vi "GV-ZoomWindowDrag.vi"(6 "Y":dbl, 7 "Gviewer in":refnum<class "Gviewer.lvclass">, 8 "error in (no error)":errorcluster, 10 "Coords":T1, 11 "pict in":picture) -> (0 "error out":errorcluster, 3 "pict out":picture)   [LabVIEW 2020, in "Sgraph_lib_V1.lvlib" / "Gviewer.lvclass"]
doc: "Andre Koelewijn, 1 May 2021\n\nDraw the zoom window"
uses:
  Gviewer.lvclass
  <vilib>/Utility/miscctls.llb/LVPoint32TypeDef.ctl
  Gviewer.lvclass/Gviewer.ctl
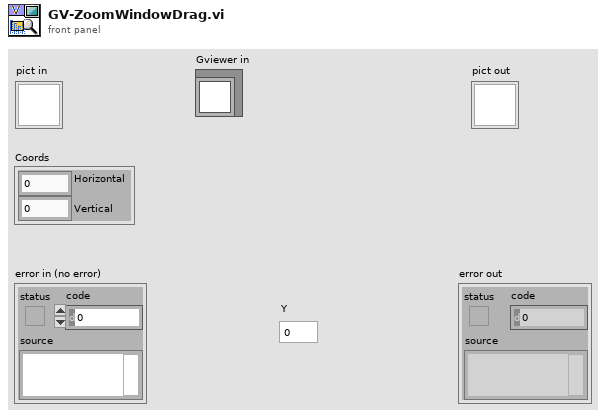
[diagram p1: front panel]
types:
  T1 = typedef "LVPoint32TypeDef.ctl" = cluster{"Horizontal":i32, "Vertical":i32}
  T2 = cluster{"Width":i16, "Style":enum32{"Solid", "Dash", "Dot", "DashDot", "DashDotDot"}}
  T3 = cluster{"left":i16, "top":i16, "right":i16, "bottom":i16}
  T4 = cluster{"horizontal":enum16{"left", "center", "right"}, "vertical":enum16{"top", "center", "bottom"}}
  T5 = typedef "Sgraph_lib_V1.lvlib/Gviewer.lvclass/Typedef_SelProperties.ctl" = cluster{"Color":u32, "LineType":T6, "max":dbl, "min":dbl}
  T6 = typedef "Sgraph_lib_V1.lvlib/Gviewer.lvclass/Typedef_LineType.ctl" = enum16{"num_bare", "num_MinMax_Area", "num_MinMax_Lines", "num_MinMax_Forfor", "num_Max_Area", "num_Max_Line", "num_Max_Forfor", "num_Min_Area", "num_Min_Line", "num_Min_Fosfor", "Boolean_Line_01", "Boolean_Area_01", "Boolean_Fosfor_01", "Boolean_Line_TF", "Boolean_Area_TF", "Boolean_Fosfor_TF", "Boolean_OnOff_Line", "Boolean_OnOff_Area", "Boolean_OnOff_Fosfor", "Boolean_spare", "StringEvent_Line", "StringEvent_TimeLine"}
  T7 = typedef "LVRectTypeDef.ctl" = cluster{"Left":i16, "Top":i16, "Right":i16, "Bottom":i16}
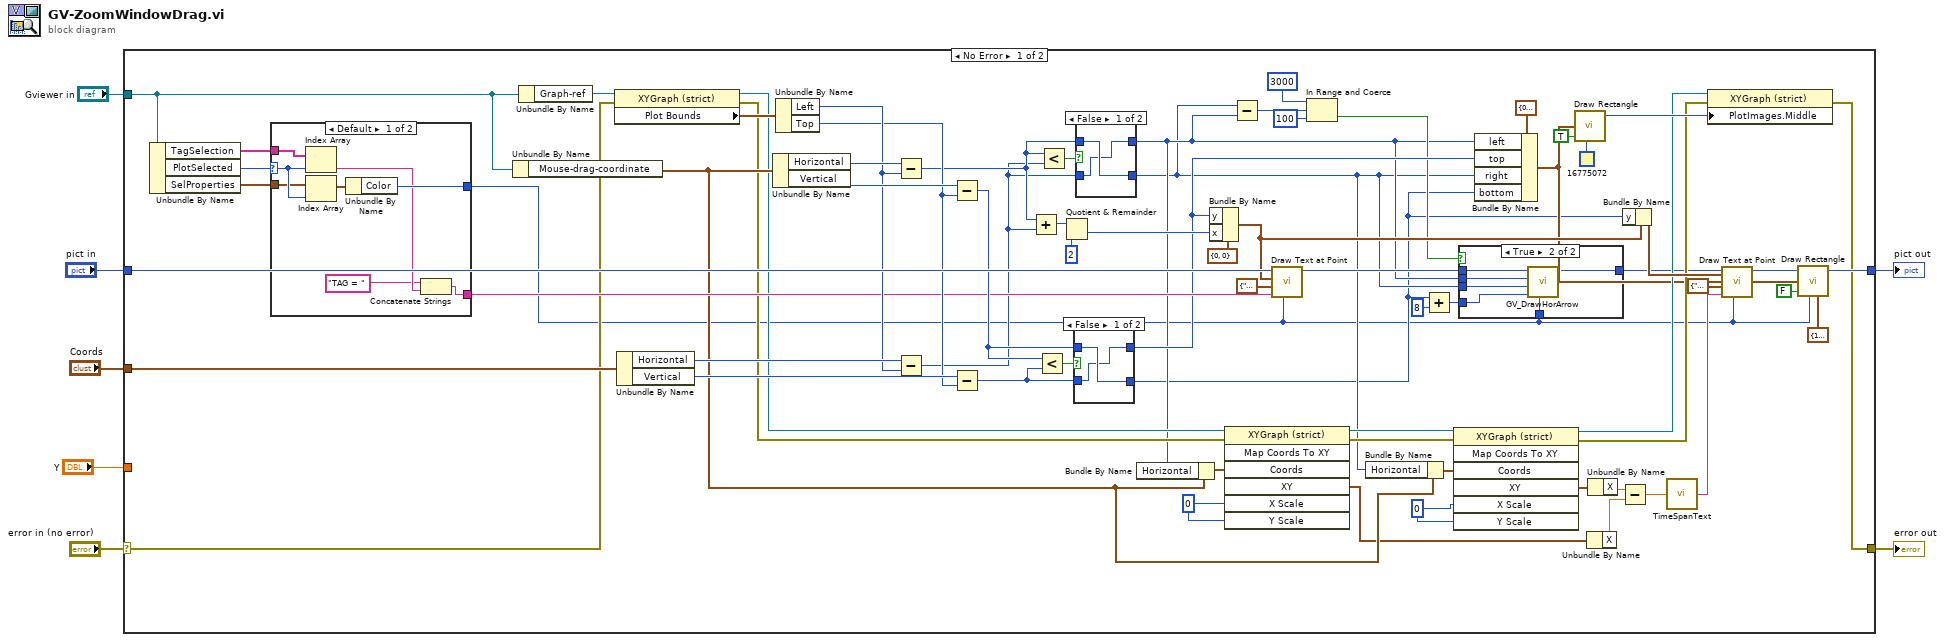
[diagram p0: block diagram]
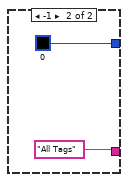
[diagram p3: hidden frame]
diagram:
  n1 = case shown="No Error" "error in (no error)" {
    selector: "error in (no error)" -> [w39 w104]
    tunnel: [w27 w104] -> w6
    tunnel: "pict in" -> [w76 w103]
    tunnel: [w55 w103] -> w4
    tunnel: "Coords" -> [w74 _]
    tunnel: "Gviewer in" -> [w51 _]
    tunnel: "Y" -> [_ _]
    frame No Error {
      w36 = 0 ("X Scale")
      w38 = 0 ("X Scale")
      n2 = Unbundle By Name(w51) -> ("TagSelection"=w53:string[], "PlotSelected"=w50:i32, "SelProperties"=w52:T5[])
      n3 = case shown="Default" w50 {
        selector: w50 -> [w89 _]
        tunnel: w53 -> [w92 _]
        tunnel: [w87 "All Tags"] -> w49
        tunnel: w52 -> [w86 _]
        tunnel: [w90 u32 0 ("Color")] -> w8
        frame Default {
          n4 = Index Array(array=w92, index=w89) -> (element=w88:string)
          n5 = Index Array(array=w86, index=w89) -> (element=w91:T5)
          n6 = Unbundle By Name(w91) -> ("Color"=w90:u32)
          n7 = Concatenate Strings("TAG = ", w88) -> (w87:string)
        }
        frame -1 {
        }
      }
      n8 = Unbundle By Name(w51) -> ("Mouse-drag-coordinate"=w34:T1)
      n9 = Unbundle By Name(w51) -> ("Graph-ref"=w69:refnum<vi>)
      n10 = property class="XYGraph (strict)"(reference=w69, error in=w39) -> (reference out=w31:refnum<vi>, error out=w29:errorcluster, "Plot Bounds"=w68:T7)
      n11 = Unbundle By Name(w74) -> ("Horizontal"=w65:i32, "Vertical"=w63:i32)
      n12 = Unbundle By Name(w34) -> ("Horizontal"=w67:i32, "Vertical"=w66:i32)
      n13 = Unbundle By Name(w68) -> ("Left"=w64:i16, "Top"=w62:i16)
      n14 = Subtract(x=w67, y=w64) -> (x-y=w48:i32)
      n15 = Subtract(x=w65, y=w64) -> (x-y=w47:i32)
      n16 = Subtract(x=w66, y=w62) -> (x-y=w60:i32)
      n17 = Subtract(x=w63, y=w62) -> (x-y=w59:i32)
      n18 = Add(x=w48, y=w47) -> (x+y=w46:i32)
      n19 = Less?(x=w60, y=w59) -> (x < y?=w58:bool)
      n20 = Less?(x=w48, y=w47) -> (x < y?=w61:bool)
      n21 = Quotient & Remainder(x=w46, y=2) -> (floor(x/y)=w43:i32)  [unwired: 1 out]
      n22 = case shown="False" w58 {
        tunnel: w60 -> [w96 w98]
        tunnel: [w95 w98] -> w42
        tunnel: [w96 w97] -> w11
        tunnel: w59 -> [w95 w97]
        frame False {
        }
        frame True {
        }
      }
      n23 = case shown="False" w61 {
        tunnel: w48 -> [w100 w102]
        tunnel: [w99 w102] -> w13
        tunnel: [w100 w101] -> w12
        tunnel: w47 -> [w99 w101]
        frame False {
        }
        frame True {
        }
      }
      n24 = Bundle By Name(cluster=w34, "Horizontal"=w13) -> (w37:T1)
      n25 = Bundle By Name(cluster=cluster{"x":i16, "y":i16} {"x"=0, "y"=0} ("origin"), "y"=w42, "x"=w43) -> (w41:cluster{"x":i16, "y":i16})
      n26 = invoke class="XYGraph (strict)" method="Map Coords To XY"(reference=w31, error in=w29, "Coords"=w37, "X Scale"=w38, "Y Scale"=w38) -> (reference out=w35:refnum<vi>, error out=w32:errorcluster, "XY"=w24:cluster{"X":dbl, "Y":dbl})  [unwired: 2 in, 4 out]
      n27 = Subtract(x=w12, y=w13) -> (x-y=w19:i32)
      n28 = call <vilib>:"Draw Text at Point.vi"("text color(black)"=w8, "text"=w49, "alignment(left, top)"=T4 {"horizontal"=enum."center", "vertical"=enum."bottom"}, "origin"=w41, "picture"=w76) -> ("new picture"=w16:picture)  [unwired: 5 in, 1 out]
      n29 = In Range and Coerce(upper limit=3000, x=w19, lower limit=100) -> (In Range?=w14:bool)  [unwired: 1 out]
      n30 = Bundle By Name(cluster=w34, "Horizontal"=w12) -> (w33:T1)
      n31 = Add(x=w11, y=8) -> (x+y=w9:i32)
      n32 = invoke class="XYGraph (strict)" method="Map Coords To XY"(reference=w35, error in=w32, "Coords"=w33, "X Scale"=w36, "Y Scale"=w36) -> (reference out=w30:refnum<vi>, error out=w28:errorcluster, "XY"=w26:cluster{"X":dbl, "Y":dbl})  [unwired: 2 in, 4 out]
      n33 = case shown="True" w14 {
        tunnel: w16 -> [w78 w84]
        tunnel: [w78 w83] -> w15
        tunnel: w13 -> [_ w82]
        tunnel: w12 -> [_ w81]
        tunnel: w9 -> [_ w80]
        tunnel: w8 -> [_ w79]
        frame False {
        }
        frame True {
          n34 = call "GV_DrawHorArrow.vi"("Color"=w79, "Vertical"=w80, "Right"=w81, "Left"=w82, "Pict-in"=w84) -> ("Pict-out"=w83:picture)  [unwired: 6 in]
        }
      }
      n35 = Bundle By Name(cluster=T3 {"left"=0, "top"=0, "right"=0, "bottom"=0} ("rect"), "left"=w13, "top"=w42, "right"=w12, "bottom"=w11) -> (w20:T3)
      n36 = call <vilib>:"Draw Rectangle.vi"("rect"=w20, "fill?(F)"=TRUE, "color(black)"=u32 16775072) -> ("new picture"=w73:picture)  [unwired: 6 in]
      n37 = Unbundle By Name(w24) -> ("X"=w23:dbl)
      n38 = Unbundle By Name(w26) -> ("X"=w25:dbl)
      n39 = Subtract(x=w25, y=w23) -> (x-y=w22:dbl)
      n40 = Bundle By Name(cluster=w41, "y"=w11) -> (w40:cluster{"x":i16, "y":i16})
      n41 = call "TimeSpanText.vi"("Timespan"=w22) -> ("TimeSpanText"=w21:string)  [unwired: 4 in]
      n42 = property class="XYGraph (strict)"(reference=w30, error in=w28, "PlotImages.Middle"=w73) -> (error out=w27:errorcluster)  [unwired: 1 out]
      n43 = call <vilib>:"Draw Text at Point.vi"("text color(black)"=w8, "text"=w21, "alignment(left, top)"=T4 {"horizontal"=enum."center", "vertical"=enum."top"}, "origin"=w40, "picture"=w15) -> ("new picture"=w56:picture)  [unwired: 5 in, 1 out]
      n44 = call <vilib>:"Draw Rectangle.vi"("picture"=w56, "rect"=w20, "fill?(F)"=FALSE, "color(black)"=w8, "pen"=T2 {"Width"=1, "Style"=enum."Dot"}) -> ("new picture"=w55:picture)  [unwired: 4 in]
    }
    frame Error {
    }
  }
  "error out" <- w6
  "pict out" <- w4
